vi "Apply Perspective.vi"(5 "File Path (Image Calibration Left)":path=path "C:/Users/whitemrj/Desktop/New folder/pizza cal.png", 7 "File Path (Image Calibration Right)":path=path "C:/Users/whitemrj/Desktop/New folder/pizza cal.png", 8 "error in":errorcluster, 9 "Left Image in":T1, 10 "Right Image in":T1) -> (0 "error out":errorcluster, 1 "Left Image out":T1, 2 "Right Image out":T1)   [LabVIEW 2012]
uses:
  <vilib>/vision/Image Controls.llb/IMAQ Image.ctl
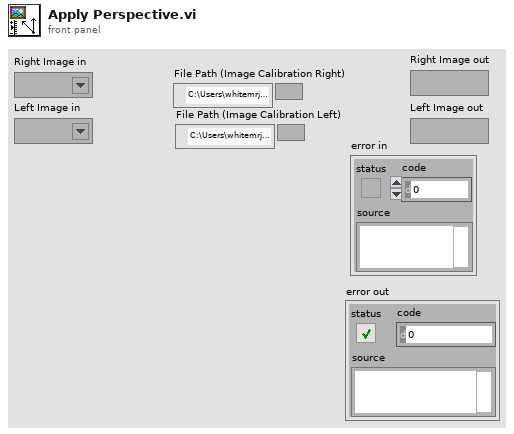
[diagram p1: front panel]
types:
  T1 = typedef "IMAQ Image.ctl" = refnum<image>
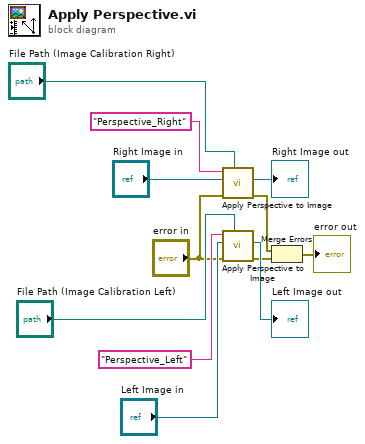
[diagram p0: block diagram]
diagram:
  n1 = call "Apply Perspective to Image.vi"("File Path (Image Calibration)"="File Path (Image Calibration Right)", "error in"="error in", "Image in"="Right Image in", "Image Name"="Perspective_Right") -> ("error out"=w2:errorcluster, "Image out"=→"Right Image out":T1)  [unwired: 6 in]
  n2 = call "Apply Perspective to Image.vi"("File Path (Image Calibration)"="File Path (Image Calibration Left)", "error in"="error in", "Image in"="Left Image in", "Image Name"="Perspective_Left") -> ("error out"=w6:errorcluster, "Image out"=→"Left Image out":T1)  [unwired: 6 in]
  n3 = Merge Errors(w2, w6) -> (→"error out":errorcluster)
